vi "P13_Toggle.vi"() -> ()   [LabVIEW 2022 SP3]
panel:
  in  "stop":bool
  in  "TMP":bool
  out "L1":bool
  in  "B1":bool
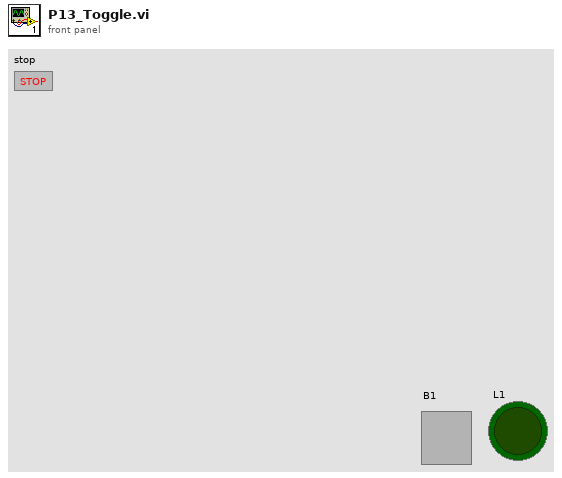
[diagram p1: front panel]
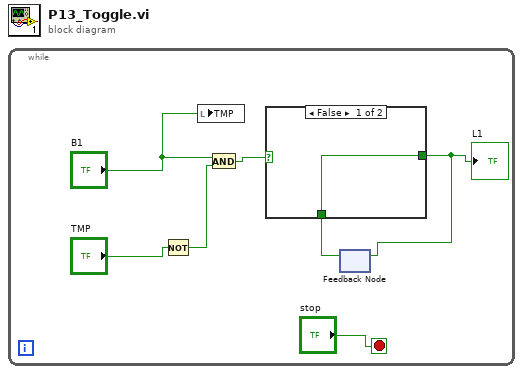
[diagram p0: block diagram]
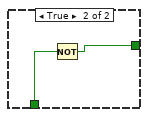
[diagram p2: hidden frame]
diagram:
  n1 = while {
    stop <- "stop" stop-if-true
    n2 = Not(x="TMP") -> (.not. x?=w7:bool)
    n3 = local write "TMP"("B1") -> ()
    n4 = And(x="B1", y=w7) -> (x .and. y?=w1:bool)
    n5 = feedback #1() -> (w2:bool)  [unwired: 1 in]
    n6 = case shown="False" w1 {
      tunnel: [w8 w9] -> w3
      tunnel: w2 -> [w8 w10]
      frame False {
      }
      frame True {
        n7 = Not(x=w10) -> (.not. x?=w9:bool)
      }
    }
    "L1" <- w3
    n8 = feedback-in #1(w3) -> ()
  }
